vi "DecideWhenToShift.vi"(4 "Force to Low Gear":bool, 6 "Force To High Gear":bool, 7 "Drive Motor Speed (rpm)":dbl, 8 "Time Below Speed (ms)":u32, 9 "Time Above Speed (ms)":u32, 10 "Switch to Low Gear (rpm)":dbl, 11 "Switch to High Gear (rpm)":dbl) -> (3 "Requested Shifter State":bool)   [LabVIEW 2023]
doc: "This VI decides when to shift a swerve module based on the drive motor RPM. Includes a hysteresis to prevent vacillation."
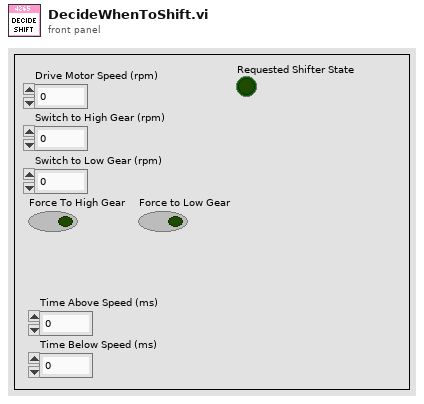
[diagram p1: front panel]
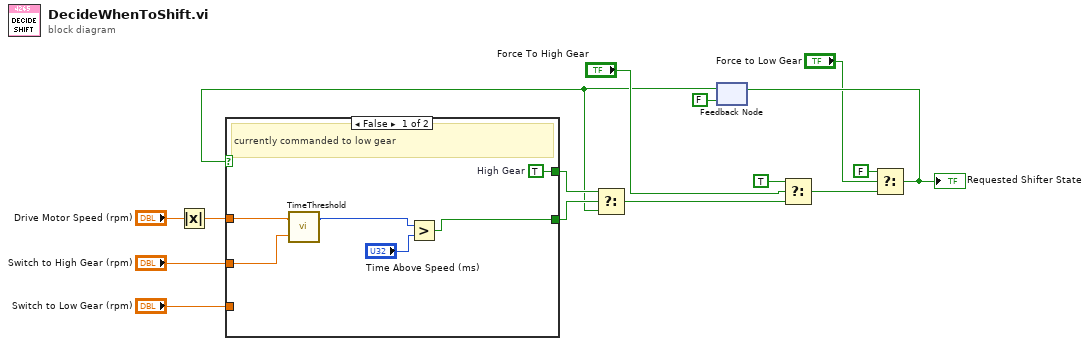
[diagram p0: block diagram]
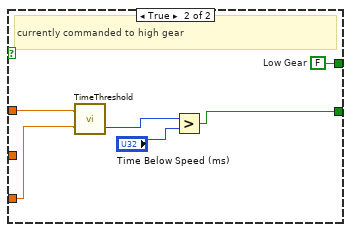
[diagram p2: hidden frame]
diagram:
  n1 = Absolute Value(x="Drive Motor Speed (rpm)") -> (abs(x)=w1:dbl)
  n2 = feedback #1(FALSE ("High Gear")) -> (w2:bool)
  n3 = case shown="False" w2 {
    tunnel: w1 -> [w18 w24]
    tunnel: "Switch to High Gear (rpm)" -> [w17 _]
    tunnel: "Switch to Low Gear (rpm)" -> [_ w23]
    tunnel: [w19 w25] -> w9
    tunnel: [w20 w26] -> w8
    frame False {
      w20 = TRUE  # High Gear
      # "currently commanded to low gear"
      n4 = call "TimeThreshold.vi"("Threshold"=w17, "Current Value"=w18) -> ("Time Above Threshold (ms)"=w16:u32)  [unwired: 1 out]
      n5 = Greater?(x=w16, y="Time Above Speed (ms)") -> (0:w19:bool)
    }
    frame True {
      w26 = FALSE  # Low Gear
      # "currently commanded to high gear"
      n6 = call "TimeThreshold.vi"("Threshold"=w23, "Current Value"=w24) -> ("Time Below Threshold (ms)"=w22:u32)  [unwired: 1 out]
      n7 = Greater?(x=w22, y="Time Below Speed (ms)") -> (0:w25:bool)
    }
  }
  n8 = Select(t=w8, s=w9, f=w2) -> (s? t:f=w6:bool)
  n9 = Select(t=TRUE, s="Force To High Gear", f=w6) -> (s? t:f=w5:bool)
  n10 = Select(t=FALSE, s="Force to Low Gear", f=w5) -> (s? t:f=w15:bool)
  "Requested Shifter State" <- w15
  n11 = feedback-in #1(w15) -> ()
